vi "Pre Analysis plugin Wing Pitch.vi"   [LabVIEW 2022 SP3]
uses:
  Controls/Time_Trace_Cluster.ctl
  Globals/Meas_global.vi
panel:
  # "Clamps Hotwire velocities outside specified range to be mean of entire signal"
types:
  T1 = typedef "Analysis_info_cluster.ctl" = cluster{"Colour":u32, "Inst type":T2, "Inst name":string, "Symbol":string, "Code name":string, "Extra Info":string, "Inst Array":T3, "Extra Titles":string[], "Extra Values":string[], "U":dbl, "u^2":dbl, "u^3":dbl, "u^4":dbl, "Skew_u":dbl, "Kurt_u":dbl, "Sd Error in Mean":dbl, "% u'/U":dbl, "X":dbl, "Y":dbl, "Z":dbl, "Timescale integral Estimate":dbl, "Sd Error in Variance":dbl, "Calib File":path, "Calib Constants":dbl[], "Output Position":bool, "Stats":enum16{"None", "Basic", "Full"}, "Av Sampling Rate":dbl, "Av No of Samples":dbl, "Total Meas Time (s)":dbl, "ADAM Ch Name":string, "Max value":dbl, "Min value":dbl, "Req Sample Rate Hz":dbl, "Sync Delay Time (s)":dbl, "Ch No":i16, "Device":string, "Use Latest Calib":bool, "Port":string, "Metadata Ch Names":string[], "Metadata Ch Values":string[], "Label":string}
  T2 = typedef "Inst_type.ctl" = enum16{"Raw voltage", "Raw with zero offsetting", "Propeller anemometer", "Pressure Transducer", "Pitot-static tube", "Hot wire", "Cross wire 1", "Cross wire 2", "Generic Linear", "Generic Polynomial", "Generic BackPoly", "Fast FID", "Thermocouple", "Cold wire", "Pulsed Wire", "LDA Vel", "LDA Tran time", "LDA Arr time", "Microphone"}
  T3 = typedef "Instrument_Array.ctl" = enum16{"PWA", "LDA", "Analogue"}
  T4 = typedef "Time_Trace_Cluster.ctl" = cluster{"Weighting":dbl[], "Voltage":dbl[], "Eng Values":dbl[]}
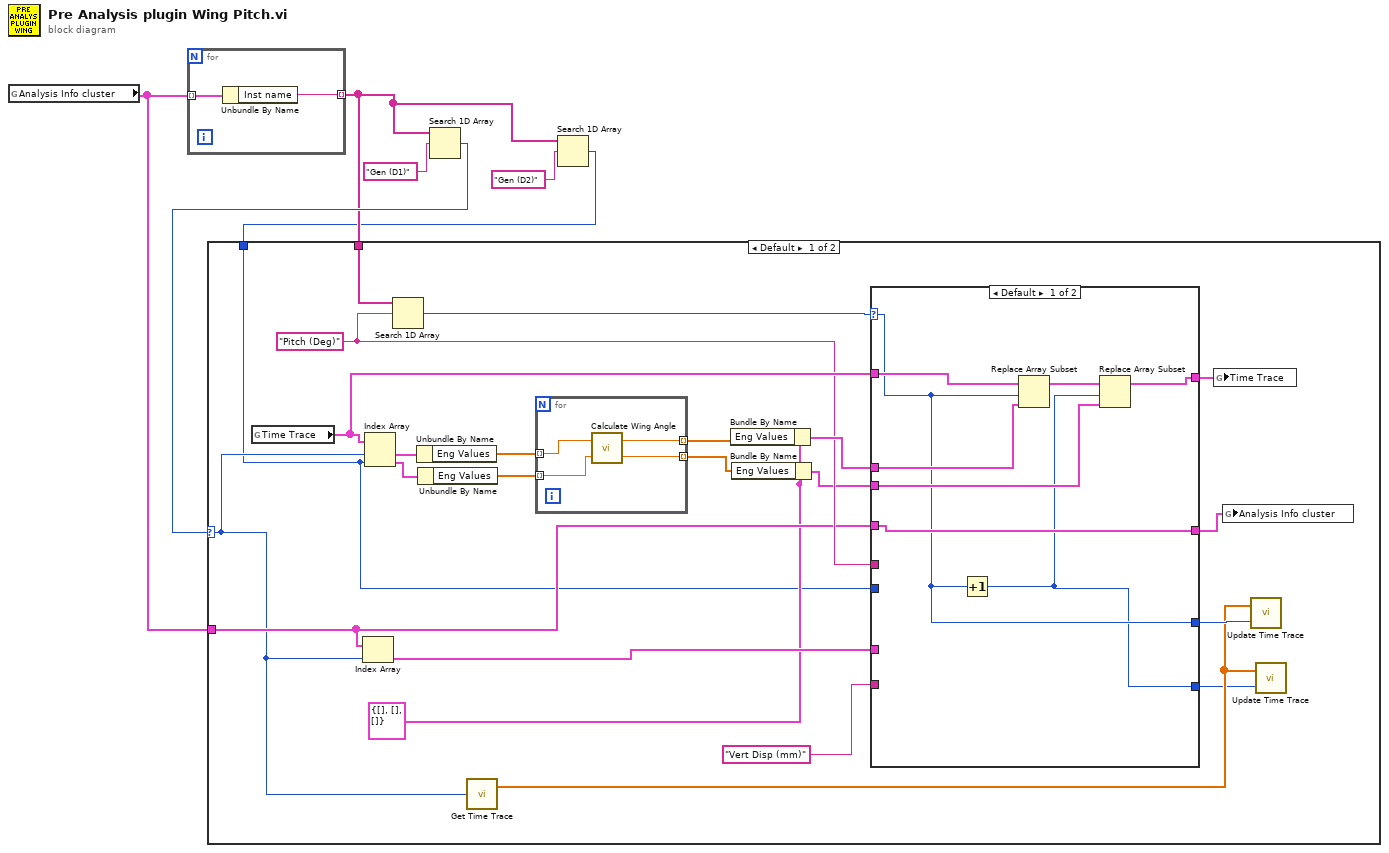
[diagram p0: block diagram]
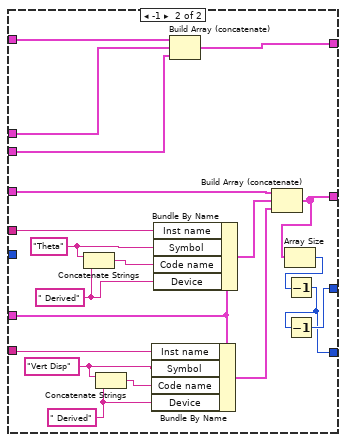
[diagram p2: hidden frame]
diagram:
  n1 = global read "Meas_global.vi" "Analysis Info cluster"() -> (w4:T1[])
  n2 = for {
    tunnel: w4 -> [w8] mode=indexing
    tunnel: [w7] -> w2 mode=indexing
    n3 = Unbundle By Name(w8) -> ("Inst name"=w7:string)
  }
  n4 = Search 1D Array(1D array=w2, element="Gen (D1)") -> (index of element=w5:i32)  [unwired: 1 in]
  n5 = Search 1D Array(1D array=w2, element="Gen (D2)") -> (index of element=w1:i32)  [unwired: 1 in]
  n6 = case shown="Default" w5 {
    selector: w5 -> [w21 _]
    tunnel: w4 -> [w23 _]
    tunnel: w2 -> [w30 _]
    tunnel: w1 -> [w11 _]
    frame Default {
      w24 = "Pitch (Deg)" ("element")
      w15 = T4 {"Weighting"=[], "Voltage"=[], "Eng Values"=[]} ("element")
      n7 = global read "Meas_global.vi" "Time Trace"() -> (w28:T4[])
      n8 = Index Array(array=w23, index=w21) -> (element=w25:T1)
      n9 = Index Array(array=w28, index #1=w21, index #2=w11) -> (element #1=w31:T4, element #2=w17:T4)
      n10 = Search 1D Array(1D array=w30, element=w24) -> (index of element=w29:i32)  [unwired: 1 in]
      n11 = Unbundle By Name(w31) -> ("Eng Values"=w19:dbl[])
      n12 = Unbundle By Name(w17) -> ("Eng Values"=w16:dbl[])
      n13 = call "Get Time Trace.vi"("Channel Index"=w21) -> ("Time (s)"=w10:dbl[])  [unwired: 1 out]
      n14 = for {
        tunnel: w19 -> [w35] mode=indexing
        tunnel: [w34] -> w18 mode=indexing
        tunnel: w16 -> [w33] mode=indexing
        tunnel: [w32] -> w14 mode=indexing
        n15 = call "Calculate Wing Angle.vi"("Laser D2"=w33, "Laser D1"=w35) -> ("Vertical Displacment of wing (mm)"=w32:dbl, "Angle of Wing"=w34:dbl)
      }
      n16 = Bundle By Name(cluster=w15, "Eng Values"=w18) -> (w27:T4)
      n17 = Bundle By Name(cluster=w15, "Eng Values"=w14) -> (w13:T4)
      n18 = case shown="Default" w29 {
        selector: w29 -> [w37 _]
        tunnel: w28 -> [w40 w63]
        tunnel: w27 -> [w42 w62]
        tunnel: [w38 w61] -> w26
        tunnel: w25 -> [_ w52]
        tunnel: w24 -> [_ w60]
        tunnel: w23 -> [w43 w56]
        tunnel: [w43 w55] -> w22
        tunnel: [w37 w45] -> w20
        tunnel: w13 -> [w41 w54]
        tunnel: "Vert Disp (mm)" ("element") -> [_ w50]
        tunnel: w11 -> [_ _]
        tunnel: [w36 w44] -> w9
        frame Default {
          n19 = Increment(x=w37) -> (x+1=w36:i32)
          n20 = Replace Array Subset(array=w40, new element=w42, index=w37) -> (w39:T4[])
          n21 = Replace Array Subset(array=w39, new element=w41, index=w36) -> (w38:T4[])
        }
        frame -1 {
          w47 = " Derived"
          w49 = "Vert Disp" ("Symbol")
          w58 = " Derived"
          w59 = "Theta" ("Symbol")
          n22 = Concatenate Strings(w59, w58) -> (w57:string)
          n23 = Concatenate Strings(w49, w47) -> (w48:string)
          n24 = Bundle By Name(cluster=w52, "Inst name"=w50, "Symbol"=w49, "Code name"=w48, "Device"=w47) -> (w51:T1)
          n25 = Bundle By Name(cluster=w52, "Inst name"=w60, "Symbol"=w59, "Code name"=w57, "Device"=w58) -> (w53:T1)
          n26 = Build Array (concatenate)(w63, w62, w54) -> (w61:T4[])
          n27 = Build Array (concatenate)(w56, w53, w51) -> (w55:T1[])
          n28 = Array Size(array=w55) -> (size(s)=w46:i32)
          n29 = Decrement(x=w46) -> (x-1=w44:i32)
          n30 = Decrement(x=w44) -> (x-1=w45:i32)
        }
      }
      n31 = global write "Meas_global.vi" "Time Trace"(w26) -> ()
      n32 = global write "Meas_global.vi" "Analysis Info cluster"(w22) -> ()
      n33 = call "Update Time Trace.vi"("Channel Index"=w20, "Time (s)"=w10) -> ()  [unwired: 1 in]
      n34 = call "Update Time Trace.vi"("Channel Index"=w9, "Time (s)"=w10) -> ()  [unwired: 1 in]
    }
    frame -1 {
    }
  }
